vi "VG_TimeOut_TRDU.vi"() -> ()   [LabVIEW 2020]
panel:
  out "TimeOut":bool
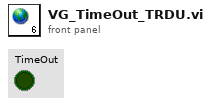
[diagram p1: front panel]
diagram:
